vi "Connect To Scanner Unit.vi"(9 "UUT Port":u32, 10 "name or relative path":string="TestScripts", 11 "Sequence path":path=path "C:/Func Jobs/SnapOn/ModisEdge/Scanner/Test Sequence/ModisEdgeScanner.seq") -> (3 "Pass":bool)   [LabVIEW 2015]
panel:
  out "standard output":string
  out "error out":errorcluster
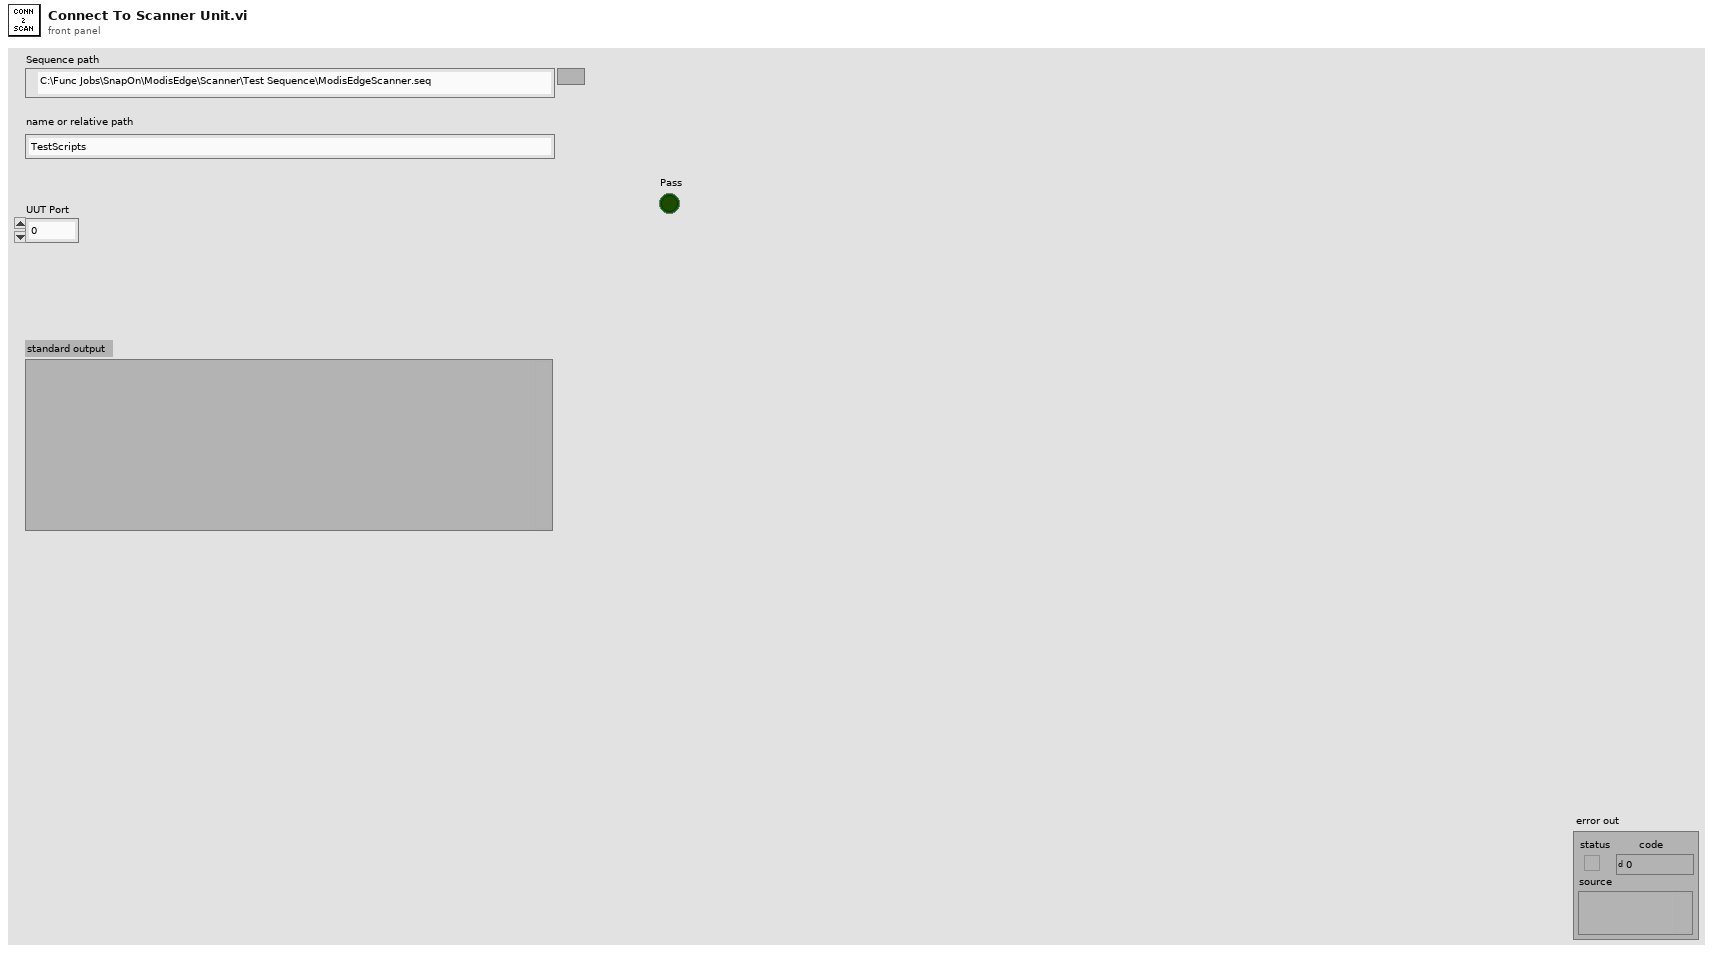
[diagram p1: front panel]
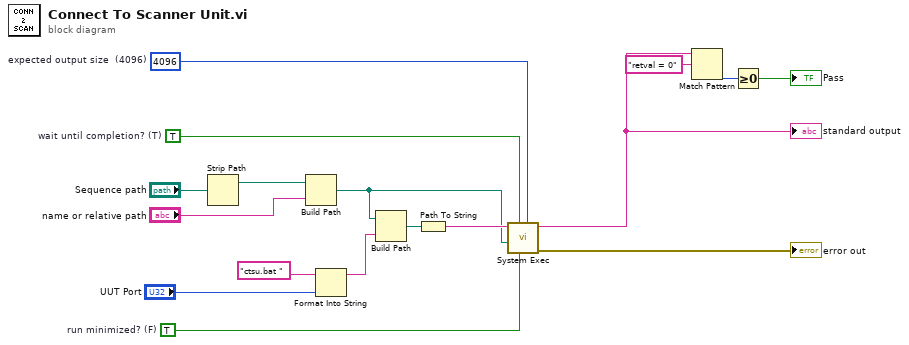
[diagram p0: block diagram]
diagram:
  w8 = TRUE  # run minimized? (F)
  w17 = TRUE  # wait until completion? (T)
  w9 = u32 4096  # expected output size  (4096)
  n1 = Strip Path(path="Sequence path") -> (stripped path=w12:path)  [unwired: 1 out]
  n2 = Build Path(base path=w12, name or relative path="name or relative path") -> (appended path=w10:path)
  n3 = Format Into String(initial string="ctsu.bat " ("Command"), "UUT Port") -> (resulting string=w1:string)  [unwired: 2 in, 1 out]
  n4 = Build Path(base path=w10, name or relative path=w1) -> (appended path=w15:path)
  n5 = Path To String(path=w15) -> (string=w14:string)
  n6 = call <vilib>:"System Exec.vi"("expected output size  (4096)"=w9, "run minimized? (F)"=w8, "wait until completion? (T)"=w17, "working directory"=w10, "command line"=w14) -> ("error out"=→"error out":errorcluster, "standard output"=w7:string)  [unwired: 3 in, 2 out]
  "standard output" <- w7
  n7 = Match Pattern(string=w7, regular expression="retval = 0") -> (offset past match=w6:i32)  [unwired: 1 in, 3 out]
  n8 = Greater Or Equal To 0?(x=w6) -> (x >= 0?=→"Pass":bool)
